vi "Write Name.vi"(8 "error in (no error)":errorcluster, 10 "Name":string, 11 "SM EOL Station Panel in":refnum<class "Panel.lvclass">) -> (0 "error out":errorcluster, 3 "SM EOL Station Panel out":refnum<class "Panel.lvclass">)   [LabVIEW 2021]
uses:
  Panel.lvclass
  C:/GitHub/SM EOL OPC Server AF/Station/Station Actor/Station.lvclass
  C:/Program Files/National Instruments/LabVIEW 2021/vi.lib/ActorFramework/Actor/Actor.lvclass
  C:/GitHub/SM EOL OPC Server AF/Station Panel/Station Panel Actor/Panel.lvclass
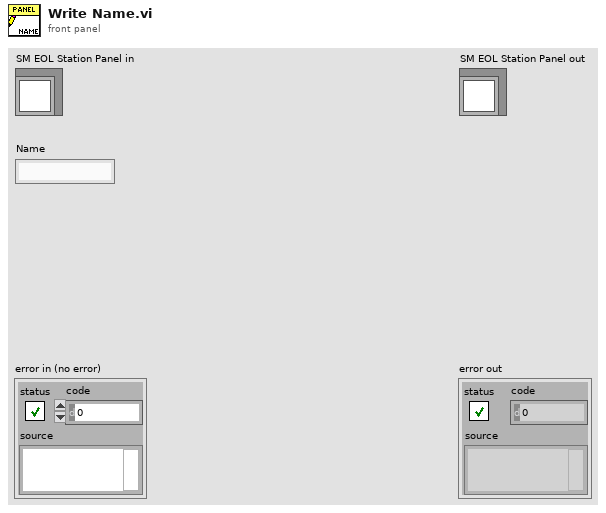
[diagram p1: front panel]
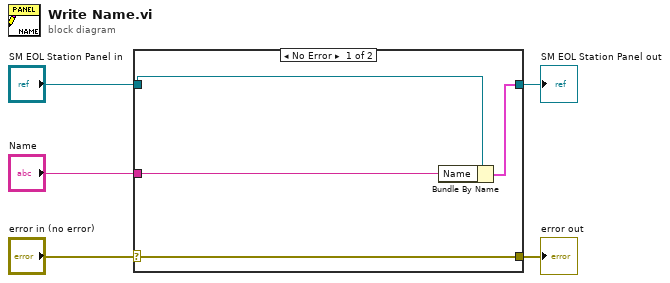
[diagram p0: block diagram]
diagram:
  n1 = case shown="No Error" "error in (no error)" {
    selector: "error in (no error)" -> [w9 w10]
    tunnel: [w9 w10] -> w4
    tunnel: [w7 w11] -> w2
    tunnel: "SM EOL Station Panel in" -> [w8 w11]
    tunnel: "Name" -> [w6 _]
    frame No Error {
      n2 = Bundle By Name(cluster=w8, "Name"=w6) -> (w7:cluster{})
    }
    frame Error {
    }
  }
  "error out" <- w4
  "SM EOL Station Panel out" <- w2
